vi "Get All Combinations of Array.vi"(8 "error in (no error)":errorcluster, 9 "Combination Length":i32, 11 "Array":variant[](array[variant])) -> (0 "error out":errorcluster, 2 "Enough Points":bool, 3 "Results Out":variant[][](array[variant]))   [LabVIEW 2016]
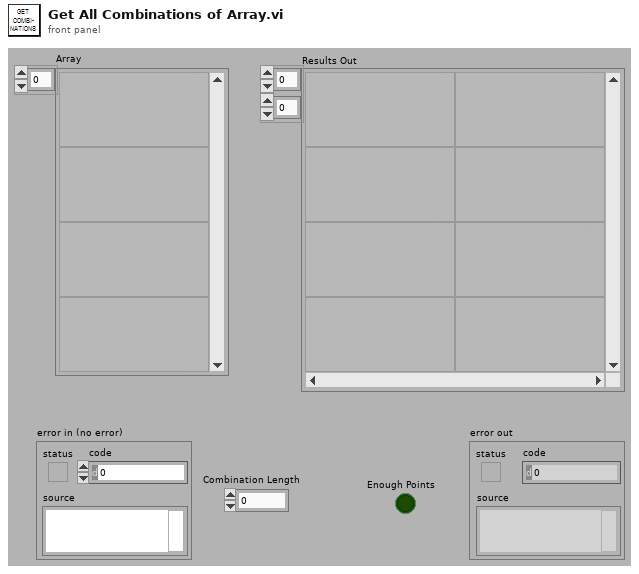
[diagram p1: front panel]
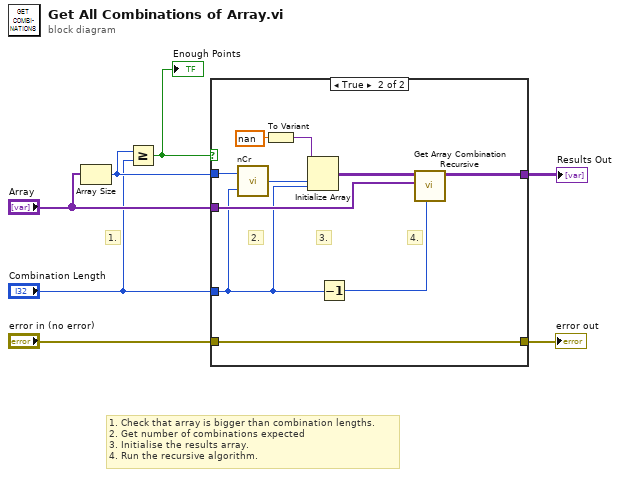
[diagram p0: block diagram]
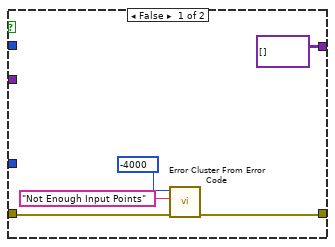
[diagram p2: hidden frame]
diagram:
  # "1. Check that array is bigger than combination lengths.\n2. Get number of combinations expected\n3. Initialise the results array.\n4. Run the recursive algorithm."
  # "1."
  n1 = Array Size(array="Array") -> (size(s)=w6:i32)
  n2 = Greater Or Equal?(x=w6, y="Combination Length") -> (x >= y?=w4:bool)
  "Enough Points" <- w4
  n3 = case shown="True" w4 {
    tunnel: "Array" -> [_ w20]
    tunnel: w6 -> [_ w18]
    tunnel: "Combination Length" -> [_ w17]
    tunnel: [w11 w16] -> w3
    tunnel: "error in (no error)" -> [w12 w16]
    tunnel: [variant[][] [] ("Results Out") w15] -> w1
    frame False {
      n4 = call <vilib>:"Error Cluster From Error Code.vi"("error in (no error)"=w12, "error message (\"\")"="Not Enough Input Points" ("error message (\"\")"), "error code (0)"=-4000) -> ("error out"=w11:errorcluster)  [unwired: 6 in]
    }
    frame True {
      # "4."
      # "3."
      # "2."
      n5 = call "nCr.vi"("R"=w17, "N"=w18) -> ("Combinations"=w22:i32)
      n6 = To Variant(anything=nan) -> (Variant=w13:variant)
      n7 = Initialize Array(w13, w22, w17) -> (w21:variant[][])
      n8 = Decrement(x=w17) -> (x-1=w19:i32)
      n9 = call "Get Array Combination Recursive.vi"("Max Column Index"=w19, "Array"=w20, "blankResultsIn"=w21) -> ("Results Out"=w15:variant[][])  [unwired: 7 in, 1 out]
    }
  }
  "error out" <- w3
  "Results Out" <- w1
